vi "process.vi"(8 "error in (no error)":errorcluster, 11 "HAL in":refnum<class "HAL.lvclass">) -> (0 "error out":errorcluster, 3 "HAL out":refnum<class "HAL.lvclass">)   [LabVIEW 2019, in "HAL.lvclass"]
uses:
  HAL.lvclass
  <vilib>/JKI/JKI SMO/SMO/SMO.lvclass
  C:/Program Files (x86)/National Instruments/LabVIEW 2019/vi.lib/JKI/JKI SMO/SMO/SMO.lvclass
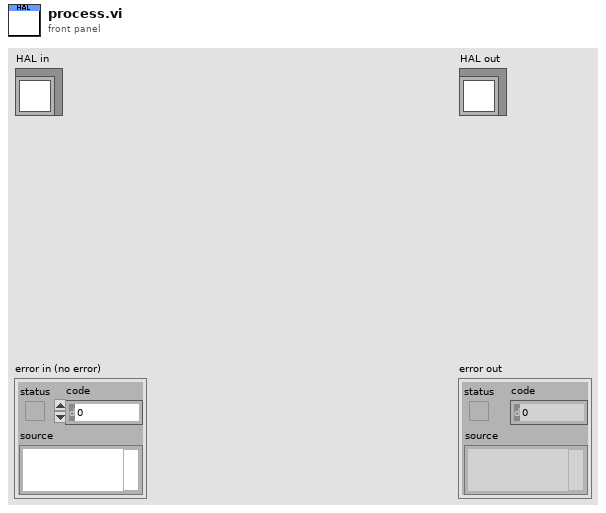
[diagram p1: front panel]
types:
  T1 = enum32{"invalid app kind", "Development System", "Run Time System", "Student Edition", "Embedded LabVIEW", "Evaluation", "Custom"}
  T2 = enum32{"Invalid", "Standard", "Closed", "Hidden", "Minimized", "Maximized"}
  T3 = cluster{"Core":cluster{"Current VI Reference":refnum<vi>, "Close Panel on Exit?":bool, "Last Error":cluster{"error":errorcluster, "previous state":string, "remaining states":string}, "Shutdown?":bool}, "SelfRef":refnum<class "HAL.lvclass">}
  T4 = cluster{"Current VI Reference":refnum<vi>, "Close Panel on Exit?":bool, "Last Error":cluster{"error":errorcluster, "previous state":string, "remaining states":string}, "Shutdown?":bool}
  T5 = typedef "SMO.lvclass/Protected Events.ctl" = cluster{"StopProcesses":refnum<user-event>, "AbortProcesses":refnum<user-event>, "Config Changed":refnum<user-event>, "Dependency":refnum<user-event>}
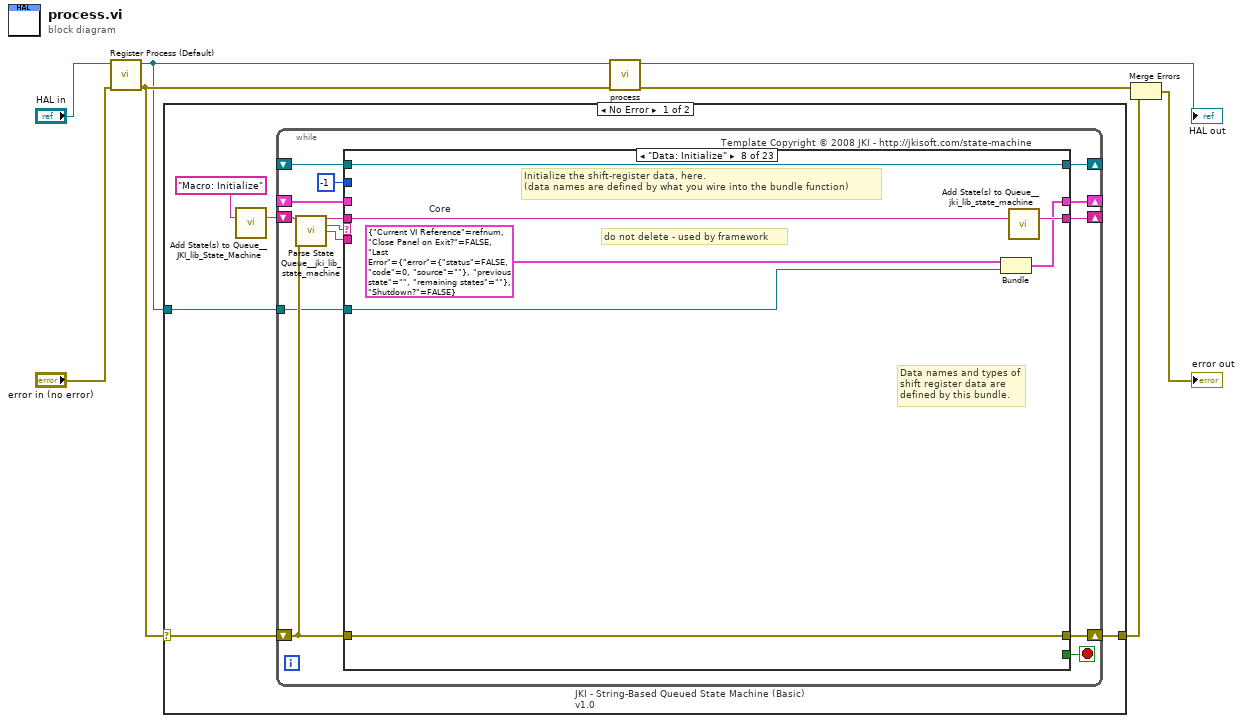
[diagram p0: block diagram]
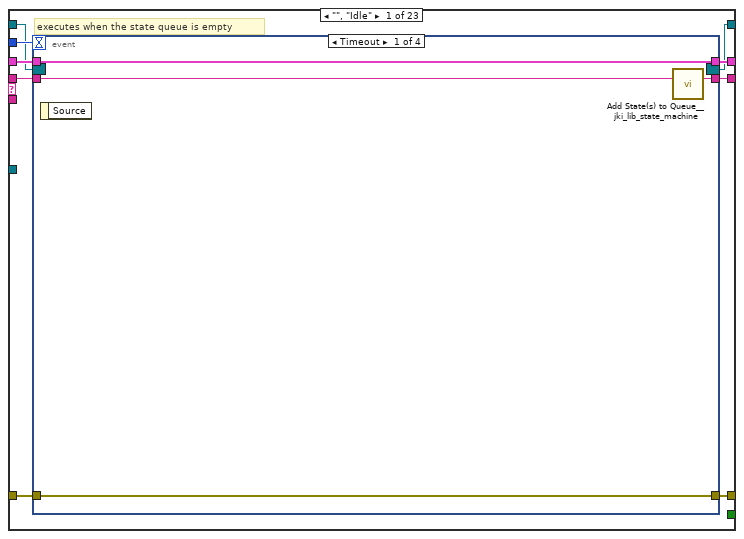
[diagram p2: hidden frame]
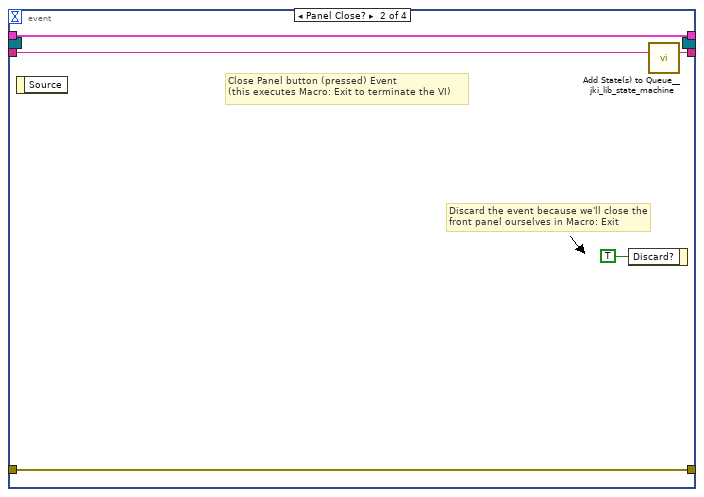
[diagram p3: hidden frame]
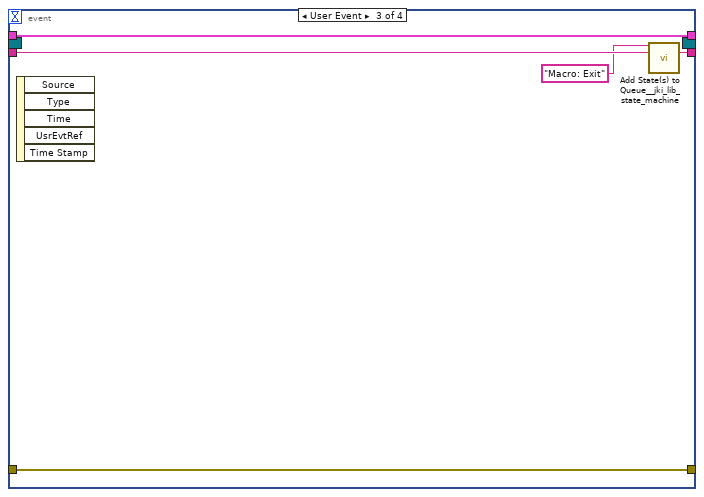
[diagram p4: hidden frame]
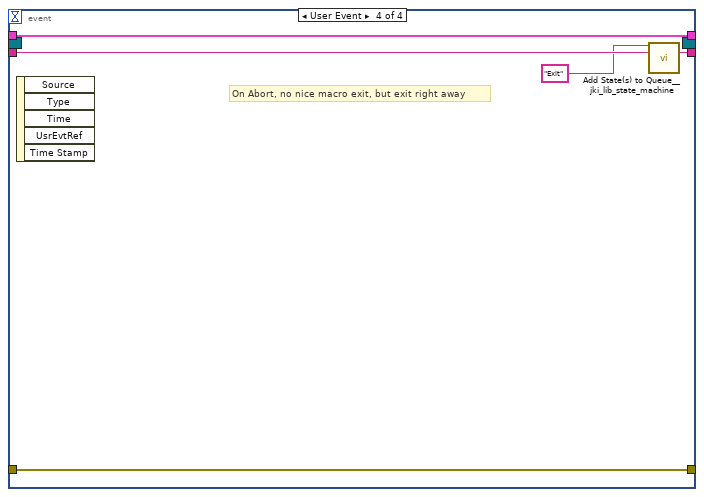
[diagram p5: hidden frame]
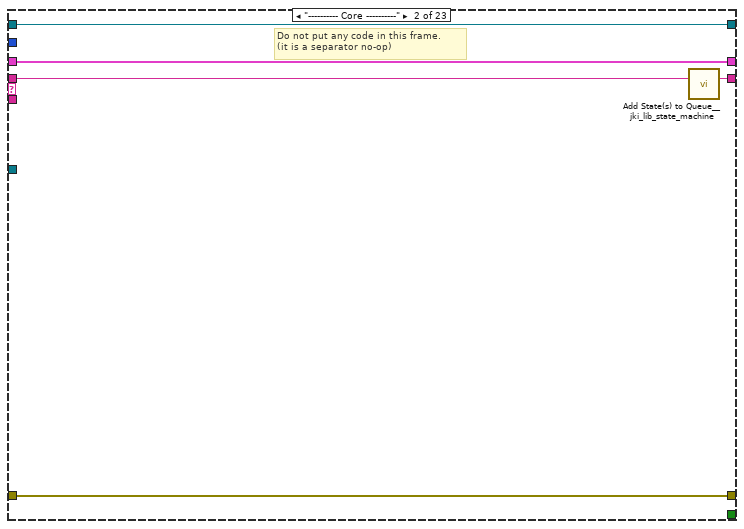
[diagram p6: hidden frame]
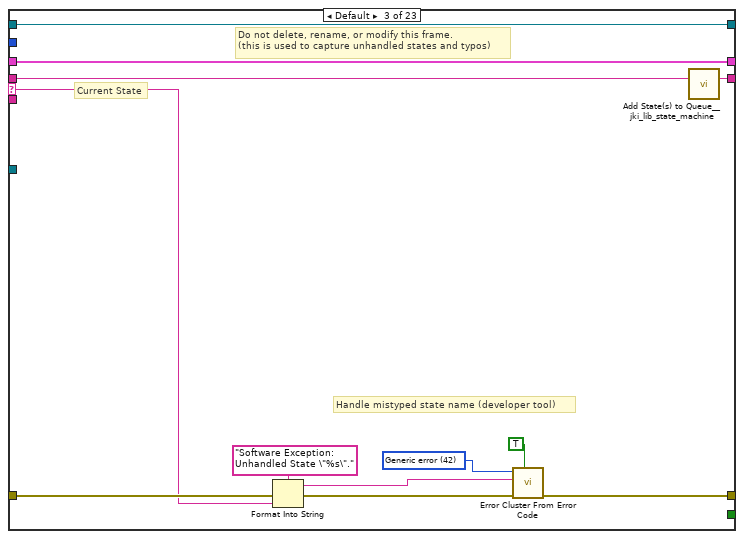
[diagram p7: hidden frame]
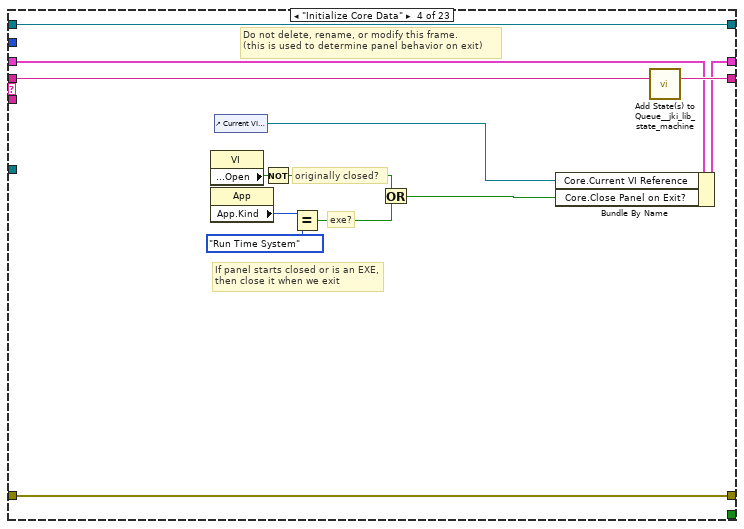
[diagram p8: hidden frame]
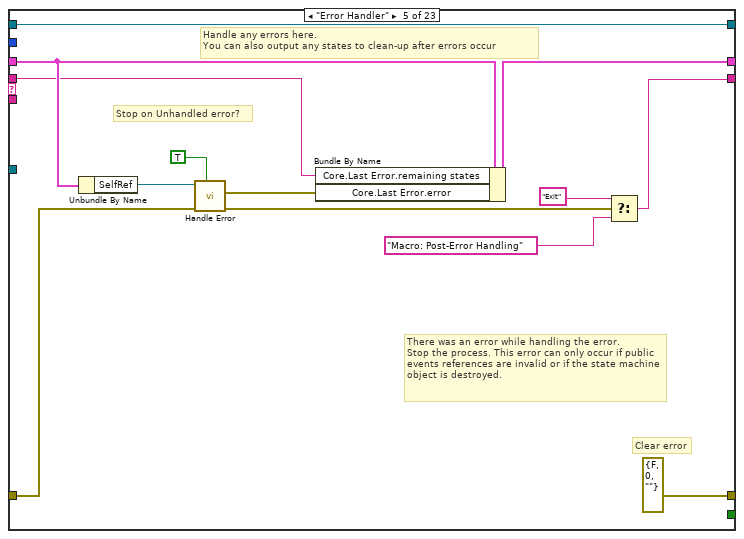
[diagram p9: hidden frame]
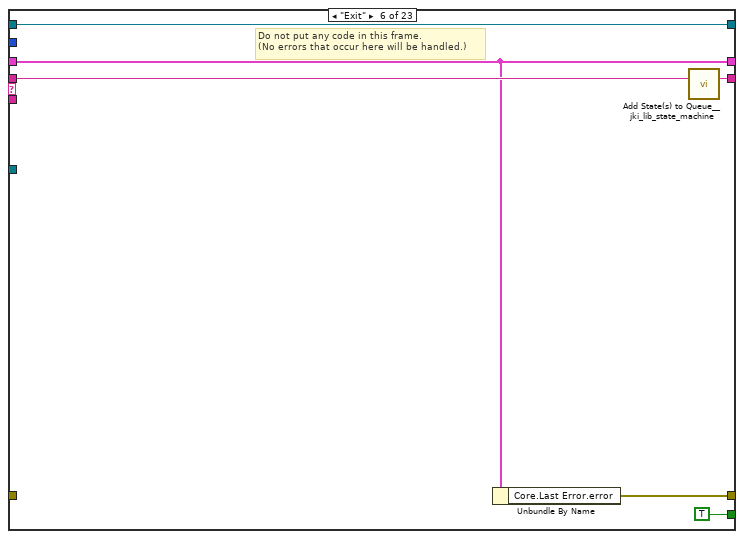
[diagram p10: hidden frame]
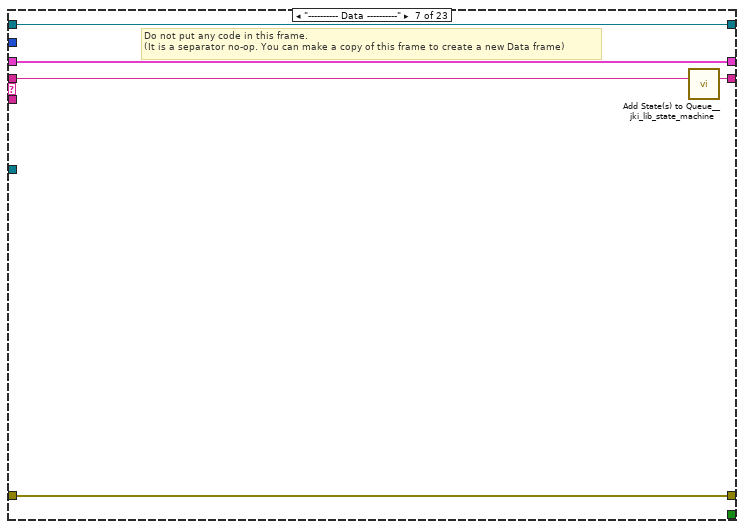
[diagram p11: hidden frame]
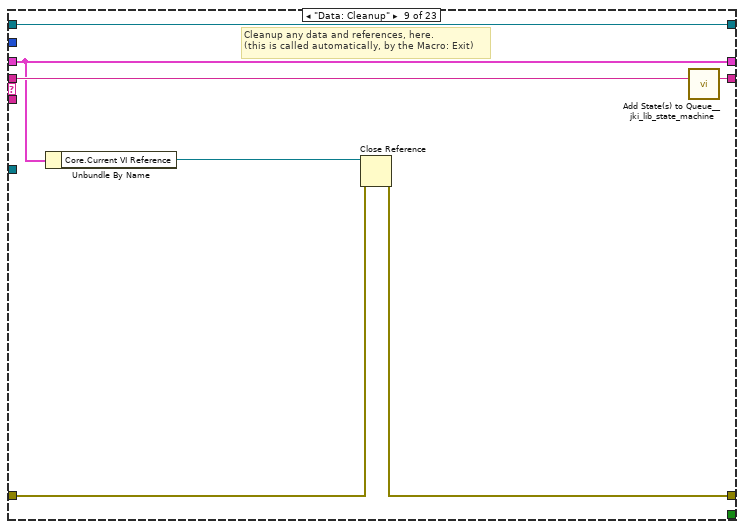
[diagram p12: hidden frame]
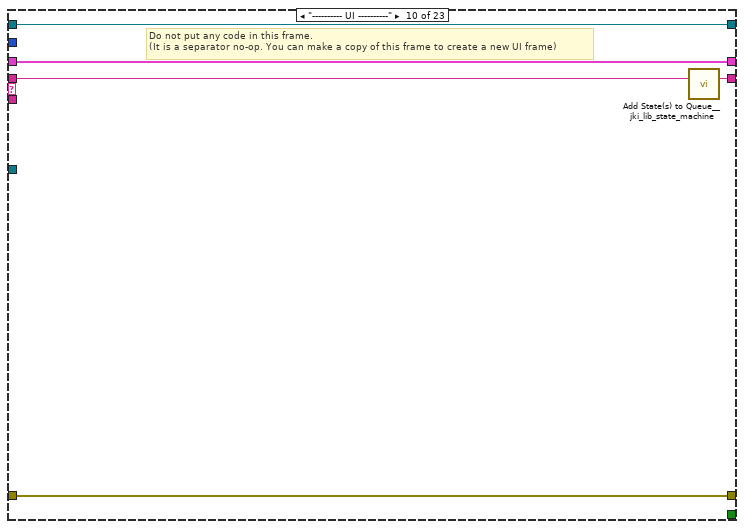
[diagram p13: hidden frame]
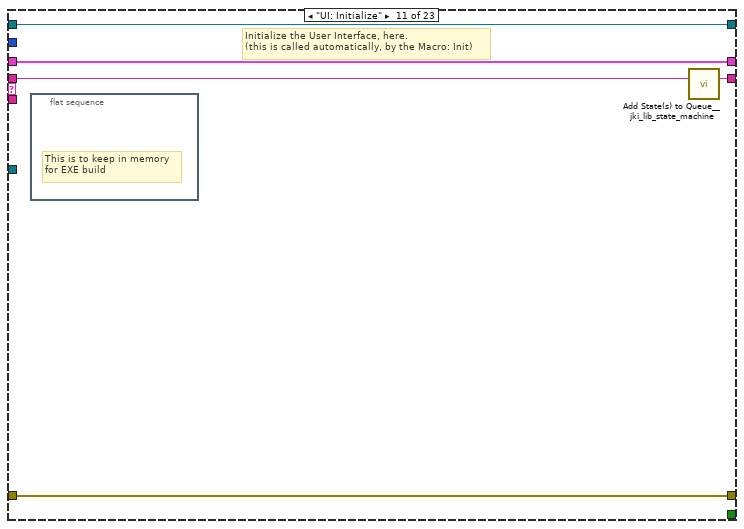
[diagram p14: hidden frame]
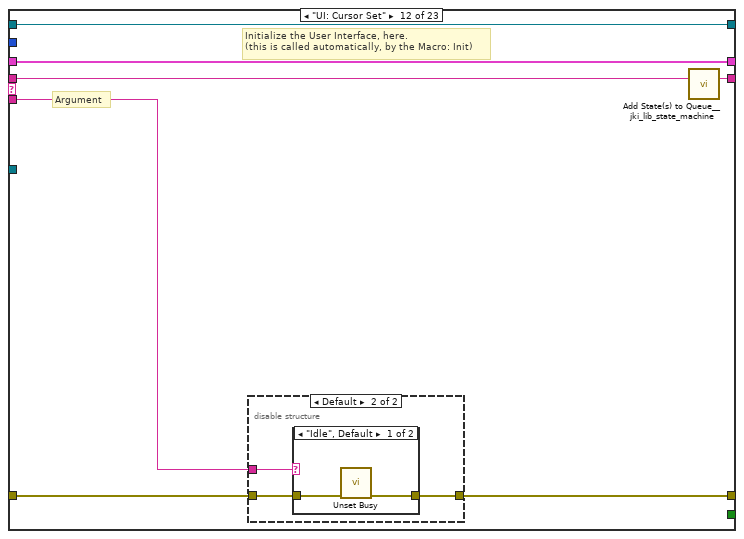
[diagram p15: hidden frame]
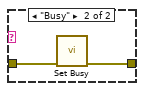
[diagram p17: hidden frame]
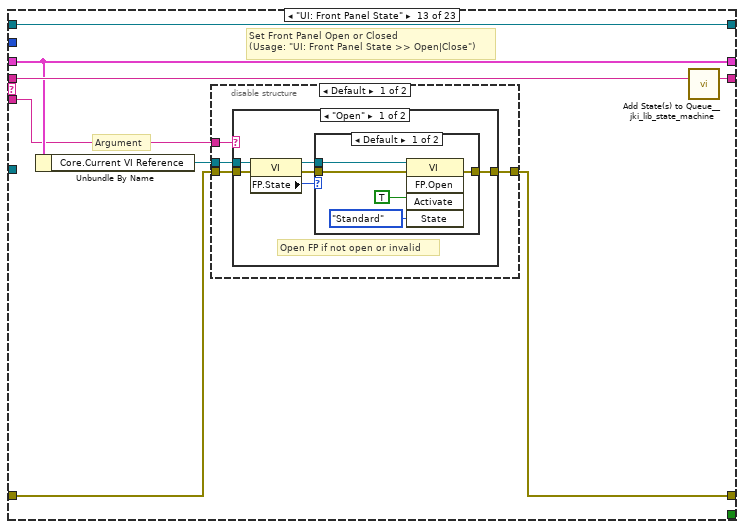
[diagram p18: hidden frame]
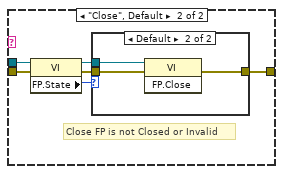
[diagram p20: hidden frame]
diagram:
  n1 = call <vilib>:"Register Process (Default).vi"("error in (no error)"="error in (no error)", "SMO"="HAL in") -> ("error out"=w8:errorcluster, "SelfRef"=w7:refnum<class "HAL.lvclass">)  [unwired: 8 in]
  n2 = case shown="No Error" w8 {
    selector: w8 -> [w12 w269]
    tunnel: w7 -> [w13 _]
    tunnel: [w11 w269] -> w5
    frame No Error {
      n3 = call <vilib>:"Add State(s) to Queue__JKI_lib_State_Machine.vi"("State(s) in (\"\")"="Macro: Initialize") -> ("States Out"=w9:string)  [unwired: 14 in]
      n4 = while "JKI - String-Based Queued State Machine (Basic) v1.0" {
        shift-right: [w20] -> _
        shift-left: _ -> [w19]
        shift-right: [w23] -> w11
        shift-left: w12 -> [w17]
        shift-right: [w22] -> _
        shift-left: w9 -> [w24]
        tunnel: w13 -> [w16]
        shift-right: [w15] -> _
        shift-left: _ -> [w14]
        stop <- w21 stop-if-true
        # "Template Copyright © 2008 JKI - http://jkisoft.com/state-machine"
        n5 = call <vilib>:"Parse State Queue__jki_lib_state_machine.vi"("State Queue"=w24, "Error In (no error)"=w17) -> ("Remaining States"=w26:string, "Current State"=w27:string, "Arguments"=w25:string)  [unwired: 11 in]
        n6 = case shown="\"Data: Initialize\"" w27 {
          selector: w27 -> [_ _ w62 _ _ _ _ _ _ _ _ _ _ _ _ _ _ _ _ _ _ _ _]
          tunnel: w26 -> [w36 w60 w66 w85 w87 w104 w109 w116 w123 w128 w133 w140 w156 w188 w197 w209 w226 w231 w242 w247 w257 w263 w268]
          tunnel: w25 -> [_ _ _ _ _ _ _ _ _ _ _ w134 w152 _ _ _ _ _ _ _ _ _ _]
          tunnel: w19 -> [w34 w57 w64 w76 w96 w100 w106 _ w118 w125 w131 w138 w154 w185 w193 w201 w216 w228 w239 w244 w255 w261 w265]
          tunnel: [w33 w58 w68 w82 errorcluster {"status"=FALSE, "code"=0, "source"=""} ("error out") w99 w107 w111 w119 w126 w130 w135 w149 w186 w195 w207 w224 w229 w233 w245 w248 w259 w266] -> w23
          tunnel: w17 -> [w32 w58 w67 w82 w93 _ w107 w111 w120 w126 w130 w136 w150 w186 w195 w207 w224 w229 w234 w245 w251 w259 w266]
          tunnel: [w35 w59 w65 w84 w86 w103 w108 w115 w122 w127 w132 w139 w155 w187 w196 w208 w225 w230 w241 w246 w256 w262 w267] -> w22
          tunnel: [_ _ _ _ _ TRUE _ _ _ _ _ _ _ _ _ _ _ _ _ _ _ _ _] -> w21
          tunnel: [w31 w57 w64 w83 w95 w100 w106 w114 w118 w125 w131 w138 w154 w185 w193 w205 w215 w228 w239 w244 w255 w261 w265] -> w20
          tunnel: -1 ("Timeout") -> [w30 _ _ _ _ _ _ _ _ _ _ _ _ _ _ _ _ _ _ _ _ _ _]
          tunnel: w16 -> [_ _ _ _ _ _ _ w110 _ _ _ _ _ _ _ _ _ _ _ _ _ _ _]
          tunnel: [w28 w56 w61 w73 w98 w101 w105 w113 w117 w124 w129 w137 w153 w184 w194 w206 w218 w227 w240 w243 w253 w260 w264] -> w15
          tunnel: w14 -> [w29 w56 w61 w73 w98 w101 w105 w113 w117 w124 w129 w137 w153 w184 w194 w206 w218 w227 w240 w243 _ w260 w264]
          frame "", "Idle" {
            # "executes when the state queue is empty"
            n7 = event shown="[0] Timeout" {
              selector: w29 -> [_ _ _ _]
              dyn-events: [_ _ _ _] -> w28
              timeout: w30 -> [_ _ _ _]
              tunnel: w36 -> [w40 w45 w50 w55]
              tunnel: [w39 w44 w49 w54] -> w35
              tunnel: w34 -> [w37 w41 w47 w52]
              tunnel: [w38 w43 w48 w53] -> w33
              tunnel: w32 -> [w38 w43 w48 w53]
              tunnel: [w37 w41 w47 w52] -> w31
              event Timeout {
                n8 = event-data() -> ()  [unwired: 1 in, 1 out]
                n9 = call <vilib>:"Add State(s) to Queue__jki_lib_state_machine.vi"("State(s) in (\"\")"=w40) -> ("States Out"=w39:string)  [unwired: 14 in]
              }
              event Panel Close? {
                # "Discard the event because we'll close the front panel ourselves in Macro: Exit"
                # "Close Panel button (pressed) Event\n(this executes Macro: Exit to terminate the VI)"
                n10 = event-data() -> ()  [unwired: 1 in, 1 out]
                n11 = event-data("Discard?"=TRUE) -> ()  [unwired: 1 in, 1 out]
                n12 = call <vilib>:"Add State(s) to Queue__jki_lib_state_machine.vi"("State(s) in (\"\")"=w45) -> ("States Out"=w44:string)  [unwired: 14 in]
              }
              event User Event {
                n13 = event-data() -> ()  [unwired: 1 in, 5 out]
                n14 = call <vilib>:"Add State(s) to Queue__jki_lib_state_machine.vi"("State(s) in Front (\"\")"="Macro: Exit", "State(s) in (\"\")"=w50) -> ("States Out"=w49:string)  [unwired: 13 in]
              }
              event User Event {
                # "On Abort, no nice macro exit, but exit right away"
                n15 = event-data() -> ()  [unwired: 1 in, 5 out]
                n16 = call <vilib>:"Add State(s) to Queue__jki_lib_state_machine.vi"("State(s) in Front (\"\")"="Exit", "State(s) in (\"\")"=w55) -> ("States Out"=w54:string)  [unwired: 13 in]
              }
            }
          }
          frame "---------- Core ----------" {
            # "Do not put any code in this frame.\n(it is a separator no-op)"
            n17 = call <vilib>:"Add State(s) to Queue__jki_lib_state_machine.vi"("State(s) in (\"\")"=w60) -> ("States Out"=w59:string)  [unwired: 14 in]
          }
          frame Default {
            w71 = 42 items=["No error", "Argument error", "Memory is full", "Out of zone", "End of file", "File already open", "Generic file I/O error", "File not found", "File permission error", "Disk is full", "Duplicate path", "Too many files open", "System feature not enabled", "Resource file not found", "Cannot add resource", "Resource not found", "Image not found", "Image memory error", "Pen does not exist", "Config type invalid", "Config token not found", "Config parse error", "Config memory error", "Bad external code format", "Bad external code offset", "External code not present", "Null window", "Destroy window error", "Null menu", "Print aborted", "Bad print record", "Print driver error", "Windows error during printing", "Memory error during printing", "Print dialog error", "Generic print error", "Invalid device refnum", "Device not found", "Device parameter error", "Device unit error", "Cannot open device", "Device call aborted", "Generic error", "Cancelled by user", "Object ID too low", "Object ID too high", "Object not in heap", "Unknown heap", "Unknown object (invalid DefProc)", "Unknown object (DefProc not in table)", "Message out of range", "Invalid (null) method", "Unknown message", "Manager call not supported", "Bad address", "Network operation in progress", "Network operation timed out", "Connection is busy", "Network attribute not supported", "Network error", "Address in use", "System out of memory", "Connection aborted", "Connection refused", "Not connected", "Already connected", "Connection closed", "Initialization error (interapplication manager)", "Bad occurrence", "Wait on unbound occurrence handler", "Occurrence queue overflow", "Datalog type conflict", "Unused", "Unrecognized type (interapplication manager)", "Memory corrupt", "Failed to make temporary DLL", "Old CIN version", "Drag socket not found", "Failed to load drop-object", "Failed to register OLE object", "Failed to release OLE object", "Format specifier type mismatch", "Unknown format specifier", "Too few format specifiers", "Too many format specifiers", "Scan failed", "Newer CIN version", "Error converting to variant", "Runtime menu error", "Password tampered", "Variant attribute not found", "Incompatible variant data type", "Event data is not available", "Event Store is not present", "Occurrence is not found", "Event Queue is not created", "Event info is not available", "Refnum passed is NULL", "Error retrieving Class GUID", "Error retrieving CoClass GUID", "Error retrieving TypeLib GUID.", "Bad built application magic bytes.", "Specific driver is different from the specific driver associated with the Logical Name.", "There is no session opened to the class driver.", "Max Error", "MAX - Error with config objects", "MAX - Error loading configuration", "MAX - Group not supported"]
            # "Current State"
            # "Do not delete, rename, or modify this frame.\n(this is used to capture unhandled states and typos)"
            # "Handle mistyped state name (developer tool)"
            n18 = Format Into String(format string="Software Exception: Unhandled State \"%s\"." ("message"), error in=w67, w62) -> (resulting string=w70:string, error out=w69:errorcluster)  [unwired: 1 in]
            n19 = call <vilib>:"Error Cluster From Error Code.vi"("show call chain? (False)"=TRUE, "error in (no error)"=w69, "error message (\"\")"=w70, "error code (0)"=w71) -> ("error out"=w68:errorcluster)  [unwired: 5 in]
            n20 = call <vilib>:"Add State(s) to Queue__jki_lib_state_machine.vi"("State(s) in (\"\")"=w66) -> ("States Out"=w65:string)  [unwired: 14 in]
          }
          frame "Initialize Core Data" {
            # "Do not delete, rename, or modify this frame.\n(this is used to determine panel behavior on exit)"
            # "originally closed?"
            # "exe?"
            # "If panel starts closed or is an EXE, then close it when we exit"
            n21 = property class="VI"() -> ("Front Panel.Open"=w81:bool)  [unwired: 2 in, 2 out]
            n22 = property class="App"() -> ("App.Kind"=w80:T1)  [unwired: 2 in, 2 out]
            n23 = control-ref of="Current VI Reference"() -> (w74:refnum<vi>)
            n24 = Not(x=w81) -> (.not. x?=w78:bool)
            n25 = Equal?(x=w80, y=T1."Run Time System" ("Application:Kind")) -> (x = y?=w77:bool)
            n26 = Or(x=w78, y=w77) -> (x .or. y?=w75:bool)
            n27 = Bundle By Name(cluster=w76, "Core.Current VI Reference"=w74, "Core.Close Panel on Exit?"=w75) -> (w83:T3)
            n28 = call <vilib>:"Add State(s) to Queue__jki_lib_state_machine.vi"("State(s) in (\"\")"=w85) -> ("States Out"=w84:string)  [unwired: 14 in]
          }
          frame "Error Handler" {
            # "Stop on Unhandled error?"
            # "There was an error while handling the error.\nStop the process. This error can only occur if public events references are invalid or if the state machine object is destroyed."
            # "Handle any errors here.\nYou can also output any states to clean-up after errors occur"
            # "Clear error"
            n29 = Unbundle By Name(w96) -> ("SelfRef"=w97:refnum<class "HAL.lvclass">)
            n30 = call-dynamic "Handle Error.vi"("Stop on Unhandled Error (T)"=TRUE, "error in"=w93, "SMO"=w97) -> ("handling error"=w91:errorcluster, "Unhandled error"=w94:errorcluster)  [unwired: 6 in, 1 out]
            n31 = Bundle By Name(cluster=w96, "Core.Last Error.remaining states"=w87, "Core.Last Error.error"=w94) -> (w95:T3)
            n32 = Select(t="Exit", s=w91, f="Macro: Post-Error Handling") -> (s? t:f=w86:string)
          }
          frame "Exit" {
            # "Do not put any code in this frame.\n(No errors that occur here will be handled.)"
            n33 = Unbundle By Name(w100) -> ("Core.Last Error.error"=w99:errorcluster)
            n34 = call <vilib>:"Add State(s) to Queue__jki_lib_state_machine.vi"("State(s) in (\"\")"=w104) -> ("States Out"=w103:string)  [unwired: 14 in]
          }
          frame "---------- Data ----------" {
            # "Do not put any code in this frame.\n(It is a separator no-op. You can make a copy of this frame to create a new Data frame)"
            n35 = call <vilib>:"Add State(s) to Queue__jki_lib_state_machine.vi"("State(s) in (\"\")"=w109) -> ("States Out"=w108:string)  [unwired: 14 in]
          }
          frame "Data: Initialize" {
            w112 = T4 {"Current VI Reference"=refnum, "Close Panel on Exit?"=FALSE, "Last Error"={"error"={"status"=FALSE, "code"=0, "source"=""}, "previous state"="", "remaining states"=""}, "Shutdown?"=FALSE}  # Core
            # "do not delete - used by framework"
            # "Data names and types of shift register data are defined by this bundle."
            # "Initialize the shift-register data, here.\n(data names are defined by what you wire into the bundle function)"
            n36 = Bundle("Core"=w112, "SelfRef"=w110) -> (w114:T3)  [unwired: 1 in]
            n37 = call <vilib>:"Add State(s) to Queue__jki_lib_state_machine.vi"("State(s) in (\"\")"=w116) -> ("States Out"=w115:string)  [unwired: 14 in]
          }
          frame "Data: Cleanup" {
            # "Cleanup any data and references, here.\n(this is called automatically, by the Macro: Exit)"
            n38 = Unbundle By Name(w118) -> ("Core.Current VI Reference"=w121:refnum<vi>)
            n39 = Close Reference(reference=w121, error in (no error)=w120) -> (error out=w119:errorcluster)
            n40 = call <vilib>:"Add State(s) to Queue__jki_lib_state_machine.vi"("State(s) in (\"\")"=w123) -> ("States Out"=w122:string)  [unwired: 14 in]
          }
          frame "---------- UI ----------" {
            # "Do not put any code in this frame.\n(It is a separator no-op. You can make a copy of this frame to create a new UI frame)"
            n41 = call <vilib>:"Add State(s) to Queue__jki_lib_state_machine.vi"("State(s) in (\"\")"=w128) -> ("States Out"=w127:string)  [unwired: 14 in]
          }
          frame "UI: Initialize" {
            # "Initialize the User Interface, here.\n(this is called automatically, by the Macro: Init)"
            n42 = flat-sequence {
              frame #0 {
                # "This is to keep in memory\nfor EXE build"
              }
            }
            n43 = call <vilib>:"Add State(s) to Queue__jki_lib_state_machine.vi"("State(s) in (\"\")"=w133) -> ("States Out"=w132:string)  [unwired: 14 in]
          }
          frame "UI: Cursor Set" {
            # "Argument"
            # "Initialize the User Interface, here.\n(this is called automatically, by the Macro: Init)"
            n44 = disable-structure shown="Default" {
              disable-tunnel: w136 -> [w141 w144]
              disable-tunnel: [w141 w143] -> w135
              disable-tunnel: w134 -> [_ w142]
              frame condition #0 {
              }
              frame condition #1 (active) {
                n45 = case shown="\"Idle\", Default" w142 {
                  tunnel: w144 -> [w146 w148]
                  tunnel: [w145 w147] -> w143
                  frame "Idle", Default {
                    n46 = call <vilib>:"Unset Busy.vi"("error in (no error)"=w146) -> ("error out"=w145:errorcluster)  [unwired: 10 in]
                  }
                  frame "Busy" {
                    n47 = call <vilib>:"Set Busy.vi"("error in (no error)"=w148) -> ("error out"=w147:errorcluster)  [unwired: 9 in, 1 out]
                  }
                }
              }
            }
            n48 = call <vilib>:"Add State(s) to Queue__jki_lib_state_machine.vi"("State(s) in (\"\")"=w140) -> ("States Out"=w139:string)  [unwired: 14 in]
          }
          frame "UI: Front Panel State" {
            # "Argument"
            # "Set Front Panel Open or Closed\n(Usage: \"UI: Front Panel State >> Open|Close\")"
            n49 = Unbundle By Name(w154) -> ("Core.Current VI Reference"=w151:refnum<vi>)
            n50 = disable-structure shown="Default" {
              disable-tunnel: w150 -> [w160 w183]
              disable-tunnel: [w159 w183] -> w149
              disable-tunnel: w151 -> [w158 _]
              disable-tunnel: w152 -> [w157 _]
              frame condition #0 (active) {
                n51 = case shown="\"Open\"" w157 {
                  tunnel: w160 -> [w164 w177]
                  tunnel: [w166 w178] -> w159
                  tunnel: w158 -> [w165 w175]
                  frame "Open" {
                    # "Open FP if not open or invalid"
                    n52 = property class="VI"(reference=w165, error in=w164) -> (reference out=w162:refnum<vi>, error out=w163:errorcluster, "FP.State"=w161:T2)
                    n53 = case shown="Default" w161 {
                      tunnel: [w169 w172] -> w166
                      tunnel: w163 -> [w168 w172]
                      tunnel: w162 -> [w167 _]
                      frame Default {
                        n54 = invoke class="VI" method="FP.Open"(reference=w167, error in=w168, "Activate"=TRUE, "State"=T2."Standard") -> (error out=w169:errorcluster)  [unwired: 1 in, 4 out]
                      }
                      frame "Invalid", "Standard" {
                      }
                    }
                  }
                  frame "Close", Default {
                    # "Close FP is not Closed or Invalid"
                    n55 = property class="VI"(reference=w175, error in=w177) -> (reference out=w174:refnum<vi>, error out=w176:errorcluster, "FP.State"=w173:T2)
                    n56 = case shown="Default" w173 {
                      tunnel: [w179 w182] -> w178
                      tunnel: w176 -> [w179 w181]
                      tunnel: w174 -> [_ w180]
                      frame "Invalid", "Closed" {
                      }
                      frame Default {
                        n57 = invoke class="VI" method="FP.Close"(reference=w180, error in=w181) -> (error out=w182:errorcluster)  [unwired: 1 in, 2 out]
                      }
                    }
                  }
                }
              }
              frame condition #1 {
              }
            }
            n58 = call <vilib>:"Add State(s) to Queue__jki_lib_state_machine.vi"("State(s) in (\"\")"=w156) -> ("States Out"=w155:string)  [unwired: 14 in]
          }
          frame "---------- Macro ----------" {
            # "Do not put any code in this frame.\n(It is a separator no-op. You can make a copy of this frame to create a new Macro frame)"
            n59 = call <vilib>:"Add State(s) to Queue__jki_lib_state_machine.vi"("State(s) in (\"\")"=w188) -> ("States Out"=w187:string)  [unwired: 14 in]
          }
          frame "Macro: Initialize" {
            w191 = "UI: Initialize\n//UI: Front Panel State >> Open"  # UI: Initialize //UI: Front Panel State >> Open
            # "Initialization Macro\n(This is called once, when the VI starts)"
            n60 = call <vilib>:"Add State(s) to Queue__jki_lib_state_machine.vi"("State(s) in Front (\"\")"="Data: Initialize\nInitialize Core Data\nEvents: Register", "State(s) in (\"\")"="Process: Sync", "State(s) at Back (\"\")"=w191) -> ("States Out"=w190:string)  [unwired: 12 in]
            n61 = call <vilib>:"Add State(s) to Queue__jki_lib_state_machine.vi"("State(s) in Front (\"\")"=w190, "State(s) in (\"\")"=w197) -> ("States Out"=w196:string)  [unwired: 13 in]
          }
          frame "Macro: Post-Error Handling" {
            # "Clear Last Error?"
            n62 = Unbundle By Name(w201) -> ("Core.Last Error.remaining states"=w199:string, "Core.Shutdown?"=w200:bool)
            n63 = Unbundle By Name(w201) -> ("Core.Last Error.error"=w204:errorcluster)
            n64 = case shown="False" FALSE {
              tunnel: w204 -> [w213 _]
              tunnel: [w213 _] -> w203
              frame False {
              }
              frame True {
              }
            }
            n65 = case shown="True" w200 {
              tunnel: w199 -> [w210 w212]
              tunnel: [w210 w211] -> w198
              frame False {
                # "These are the remaining states (at the moment the error occured). States can be altered according to business logic."
                # "NOT SHUTTING DOWN"
              }
              frame True {
                # "Developer can decide to alter the states but should be aware that during the shutdown process, there are certain states that must be run for the SMO to properly shut itself (and this process) down. As such, one can add states to perform additional clean-ups, but should append the remaining state to be executed."
                # "SHUTTING DOWN"
                n66 = call <vilib>:"Add State(s) to Queue__jki_lib_state_machine.vi"("State(s) in (\"\")"=w212) -> ("States Out"=w211:string)  [unwired: 14 in]
              }
            }
            n67 = Bundle By Name(cluster=w201, "Core.Last Error.error"=w203) -> (w205:T3)
            n68 = call <vilib>:"Add State(s) to Queue__jki_lib_state_machine.vi"("State(s) in Front (\"\")"=w198, "State(s) in (\"\")"=w209) -> ("States Out"=w208:string)  [unwired: 13 in]
          }
          frame "Macro: Exit" {
            # "Exit Macro\n(This is called once, when the VI exits)"
            n69 = Unbundle By Name(w216) -> ("Core.Close Panel on Exit?"=w223:bool)
            n70 = Bundle By Name(cluster=w216, "Core.Shutdown?"=TRUE) -> (w215:T3)
            n71 = Select(t="UI: Front Panel State >> Close", s=w223, f="") -> (s? t:f=w220:string)
            n72 = call <vilib>:"Add State(s) to Queue__jki_lib_state_machine.vi"("State(s) in (\"\")"=w220, "State(s) at Back (\"\")"="Data: Cleanup\nEvents: Unregister\nProcess: Sync\nExit") -> ("States Out"=w219:string)  [unwired: 13 in]
            n73 = call <vilib>:"Add State(s) to Queue__jki_lib_state_machine.vi"("State(s) in Front (\"\")"=w219, "State(s) in (\"\")"=w226) -> ("States Out"=w225:string)  [unwired: 13 in]
          }
          frame "---------- Process ----------" {
            # "Template Separator\n(You can make a copy of, or modify, this frame)"
            n74 = call <vilib>:"Add State(s) to Queue__jki_lib_state_machine.vi"("State(s) in (\"\")"=w231) -> ("States Out"=w230:string)  [unwired: 14 in]
          }
          frame "Process: Sync" {
            n75 = Unbundle By Name(w239) -> ("SelfRef"=w235:refnum<class "HAL.lvclass">)
            n76 = call <vilib>:"WaitOnProcessSync.vi"("error in (no error)"=w234, "SMO"=w235) -> ("error out"=w233:errorcluster, "Don't run?"=w238:bool)  [unwired: 7 in, 1 out]
            n77 = Select(t="Data: Cleanup\nEvents: Unregister\nExit", s=w238, f="") -> (s? t:f=w232:string)
            n78 = call <vilib>:"Add State(s) to Queue__jki_lib_state_machine.vi"("State(s) in Front (\"\")"=w232, "State(s) in (\"\")"=w242) -> ("States Out"=w241:string)  [unwired: 13 in]
          }
          frame "---------- Events ----------" {
            # "Template Separator\n(You can make a copy of, or modify, this frame)"
            n79 = call <vilib>:"Add State(s) to Queue__jki_lib_state_machine.vi"("State(s) in (\"\")"=w247) -> ("States Out"=w246:string)  [unwired: 14 in]
          }
          frame "Events: Register" {
            n80 = Unbundle By Name(w255) -> ("SelfRef"=w252:refnum<class "HAL.lvclass">)
            n81 = call <vilib>:"GetProtectedEvents.vi"("error in (no error)"=w251, "SMO"=w252) -> ("error out"=w250:errorcluster, "SMO Protected Events"=w254:T5)  [unwired: 7 in, 1 out]
            n82 = register-events(w254) -> (reference out=w253:refnum<event-registration>, error out=w249:errorcluster)  [unwired: 2 in]
            n83 = call <vilib>:"Add State(s) to Queue__jki_lib_state_machine.vi"("State(s) in (\"\")"=w257) -> ("States Out"=w256:string)  [unwired: 14 in]
            n84 = Merge Errors(w250, w249) -> (w248:errorcluster)
          }
          frame "Events: Unregister" {
            n85 = Unregister For Events(event registration refnum=w260, error in=w259) -> (error out=w258:errorcluster)
            n86 = call <vilib>:"Clear Errors.vi"("error in (no error)"=w258) -> ()  [unwired: 5 in, 2 out]
            n87 = call <vilib>:"Add State(s) to Queue__jki_lib_state_machine.vi"("State(s) in (\"\")"=w263) -> ("States Out"=w262:string)  [unwired: 14 in]
          }
          frame "--------- Section ---------" {
            # "Section Separator\n(You can make a copy of, or modify, this frame)"
            n88 = call <vilib>:"Add State(s) to Queue__jki_lib_state_machine.vi"("State(s) in (\"\")"=w268) -> ("States Out"=w267:string)  [unwired: 14 in]
          }
        }
      }
    }
    frame Error {
    }
  }
  n89 = call-parent "process.vi"("error in"=w8, "SMO"=w7) -> ("error out"=w4:errorcluster, "SMO out"=→"HAL out":refnum<class "HAL.lvclass">)  [unwired: 8 in]
  n90 = Merge Errors(w4, w5) -> (→"error out":errorcluster)
